vi "Common-AlertHandler.vi"(6 "备注":string, 8 "报警详情":string, 9 "报警系统":string(combo), 10 "试验ID":u32, 11 "报警级别":string(combo)) -> ()   [LabVIEW 2014]
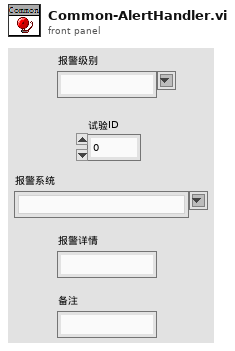
[diagram p1: front panel]
types:
  T1 = cluster{"试验ID":u32, "报警级别":string, "报警系统":string, "报警详情":string, "备注":string}
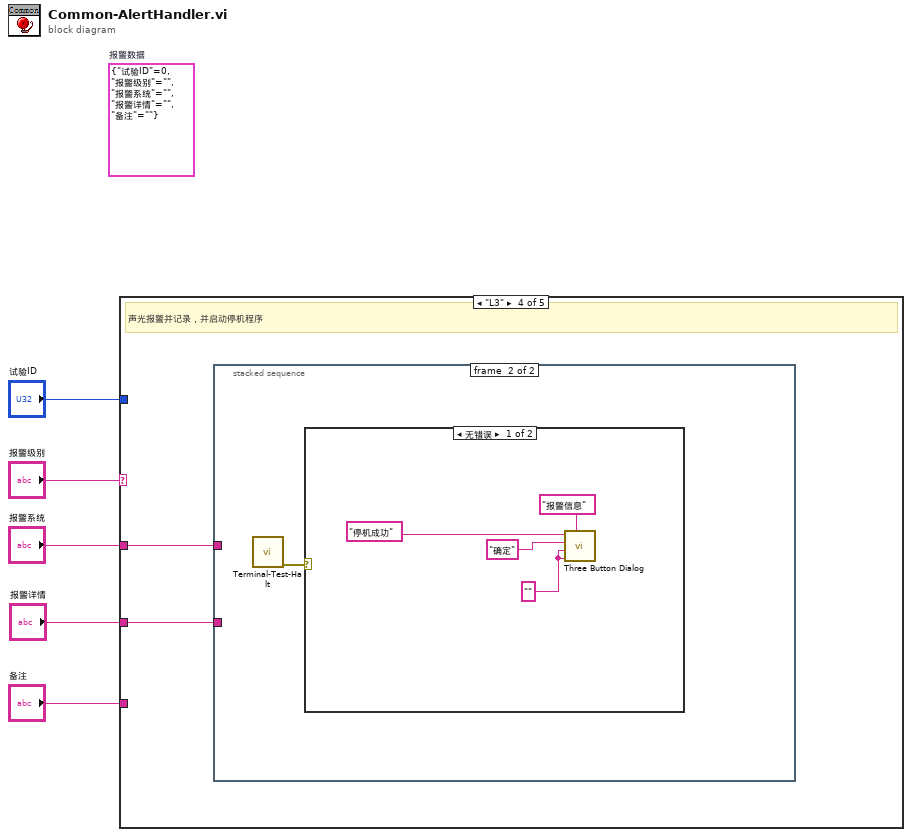
[diagram p0: block diagram]
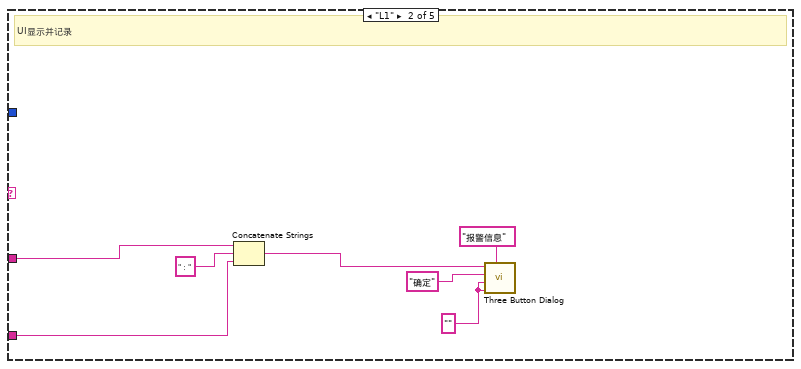
[diagram p3: hidden frame]
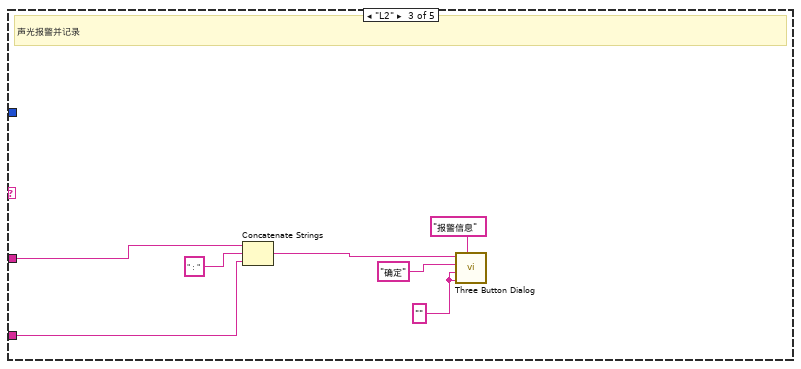
[diagram p4: hidden frame]
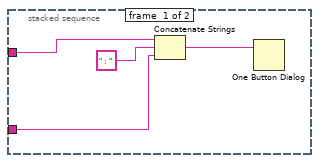
[diagram p5: hidden frame]
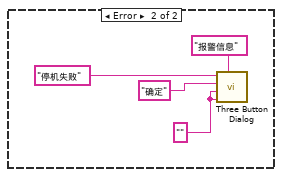
[diagram p6: hidden frame]
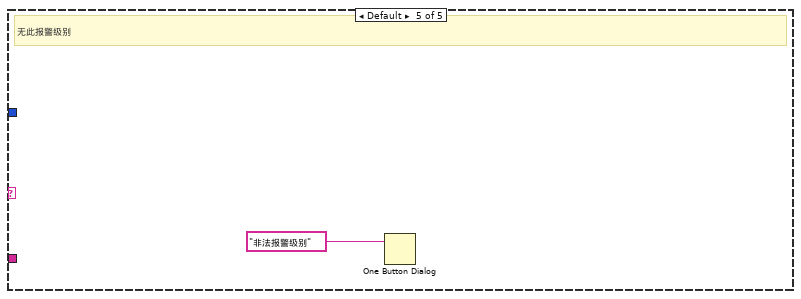
[diagram p7: hidden frame]
diagram:
  (unwired) T1 {"试验ID"=0, "报警级别"="", "报警系统"="", "报警详情"="", "备注"=""}  # 报警数据
  n1 = case shown="\"L3\"" "报警级别" {
    tunnel: "试验ID" -> [_ _ _ _ _]
    tunnel: "报警系统" -> [_ w12 w18 w21 _]
    tunnel: "报警详情" -> [_ w10 w17 w20 _]
    tunnel: "备注" -> [_ _ _ _ _]
    frame "L0" {
      # "不报警"
    }
    frame "L1" {
      w7 = "" ("Center Button Text (\"No\")")
      # "UI显示并记录"
      n2 = Concatenate Strings(w12, "：" ("字符串"), w10) -> (w9:string)
      n3 = call <vilib>:"Three Button Dialog.vi"("Window Title (\"\")"="报警信息" ("Window Title (\"\")"), "Right Button Text (\"Cancel\")"=w7, "Center Button Text (\"No\")"=w7, "Left Button Text (\"Yes\")"="确定" ("Left Button Text (\"Yes\")"), "message"=w9) -> ()  [unwired: 6 in, 1 out]
    }
    frame "L2" {
      w15 = "" ("Center Button Text (\"No\")")
      # "声光报警并记录"
      n4 = Concatenate Strings(w18, "：" ("字符串"), w17) -> (w13:string)
      n5 = call <vilib>:"Three Button Dialog.vi"("Window Title (\"\")"="报警信息" ("Window Title (\"\")"), "Right Button Text (\"Cancel\")"=w15, "Center Button Text (\"No\")"=w15, "Left Button Text (\"Yes\")"="确定" ("Left Button Text (\"Yes\")"), "message"=w13) -> ()  [unwired: 6 in, 1 out]
    }
    frame "L3" {
      # "声光报警并记录，并启动停机程序"
      n6 = stacked-sequence {
        tunnel: w21 -> [w23 _]
        tunnel: w20 -> [w22 _]
        frame #0 {
          n7 = Concatenate Strings(w23, "：" ("字符串"), w22) -> (w24:string)
          n8 = One Button Dialog(message=w24) -> ()  [unwired: 1 in, 1 out]
        }
        frame #1 {
          n9 = call "Terminal-Test-Halt.vi"() -> ("error out"=w26:errorcluster)  [unwired: 11 in]
          n10 = case shown="无错误" w26 {
            frame No Error {
              w29 = "" ("Center Button Text (\"No\")")
              n11 = call <vilib>:"Three Button Dialog.vi"("Window Title (\"\")"="报警信息" ("Window Title (\"\")"), "Right Button Text (\"Cancel\")"=w29, "Center Button Text (\"No\")"=w29, "Left Button Text (\"Yes\")"="确定" ("Left Button Text (\"Yes\")"), "message"="停机成功" ("消息")) -> ()  [unwired: 6 in, 1 out]
            }
            frame Error {
              w33 = "" ("Center Button Text (\"No\")")
              n12 = call <vilib>:"Three Button Dialog.vi"("Window Title (\"\")"="报警信息" ("Window Title (\"\")"), "Right Button Text (\"Cancel\")"=w33, "Center Button Text (\"No\")"=w33, "Left Button Text (\"Yes\")"="确定" ("Left Button Text (\"Yes\")"), "message"="停机失败" ("消息")) -> ()  [unwired: 6 in, 1 out]
            }
          }
        }
      }
    }
    frame Default {
      # "无此报警级别"
      n13 = One Button Dialog(message="非法报警级别" ("消息")) -> ()  [unwired: 1 in, 1 out]
    }
  }
